vi "M14_IMU_Hardware_Globals.vi"() -> ()   [LabVIEW 2019]
panel:
  in  "IMU":string="IMU"
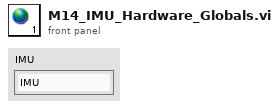
[diagram p1: front panel]
diagram:
